vi "BuildCall.vi"(7 "PythonConverter_BD in":refnum<class "PyConvBD.lvclass">, 8 "error in":errorcluster, 11 "Constant in":refnum<class "Constant.lvclass">) -> (0 "error out":errorcluster, 3 "Constant out":refnum<class "Constant.lvclass">, 5 "PythonConverter_BD out":refnum<class "PyConvBD.lvclass">)   [LabVIEW 2014, in "Constant.lvclass"]
uses:
  Constant.lvclass
  Python/PythonConverter_BD/PyConvBD.lvclass
  Python/PythonConverter_BD/TypeDefs/NodeCall_TD.ctl
  Terminal/Terminal.lvclass
  Python/Parsing/Python Functions.lvlib
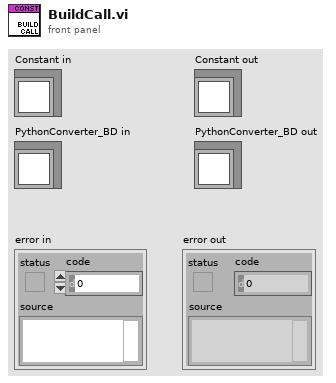
[diagram p1: front panel]
types:
  T1 = typedef "NodeCall_TD.ctl" = cluster{"call":string, "collect":string, "Threaded":bool, "branches":string[]}
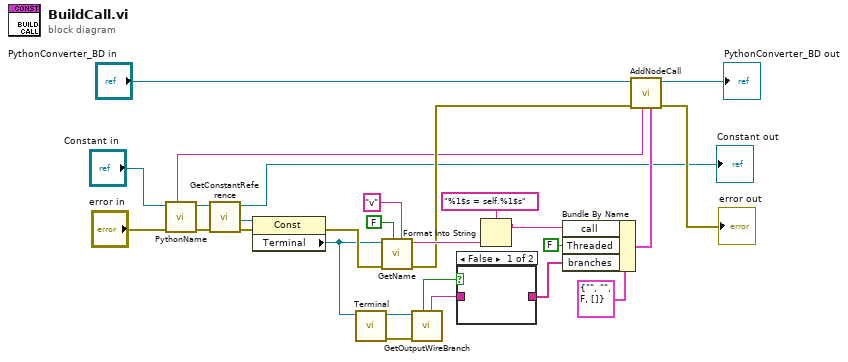
[diagram p0: block diagram]
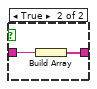
[diagram p2: hidden frame]
diagram:
  n1 = call-dynamic "PythonName.vi"("error in"="error in", "Constant in"="Constant in") -> ("error out"=w14:errorcluster, "Constant out"=w15:refnum<class "Constant.lvclass">, "UID"=w12:string)  [unwired: 6 in, 1 out]
  n2 = call "GetConstantReference.vi"("error in"=w14, "Constant in"=w15) -> ("error out"=w18:errorcluster, "reference out"=w17:refnum<vi>, "Constant out"=→"Constant out":refnum<class "Constant.lvclass">)  [unwired: 5 in]
  n3 = property class="Const"(reference=w17, error in=w18) -> (error out=w19:errorcluster, "Terminal"=w6:refnum<vi>)  [unwired: 1 out]
  n4 = call "Terminal.vi"("refnum"=w6) -> ("error out"=w4:errorcluster, "terminal"=w5:refnum<class "Terminal.lvclass">)  [unwired: 9 in]
  n5 = call "GetName.vi"("base name"="v", "add self"=FALSE, "error in"=w19, "GObj Refnum"=w6) -> ("error out"=w20:errorcluster, "name"=w23:string)  [unwired: 5 in, 1 out]
  n6 = call-dynamic "GetOutputWireBranch.vi"("error in"=w4, "Terminal in"=w5) -> ("branches"=w3:string, "branched"=w1:bool)  [unwired: 4 in, 2 out]
  n7 = case shown="False" w1 {
    tunnel: w3 -> [_ w29]
    tunnel: [_ w28] -> w2
    frame False {
    }
    frame True {
      n8 = Build Array(w29) -> (w28:string[])
    }
  }
  n9 = Format Into String(format string="%1$s = self.%1$s", w23) -> (resulting string=w9:string)  [unwired: 2 in, 1 out]
  n10 = Bundle By Name(cluster=T1 {"call"="", "collect"="", "Threaded"=FALSE, "branches"=[]} ("call"), "call"=w9, "Threaded"=FALSE, "branches"=w2) -> (w8:T1)
  n11 = call "AddNodeCall.vi"("call"=w8, "name"=w12, "error in"=w20, "PythonConverter_BD in"="PythonConverter_BD in") -> ("error out"=→"error out":errorcluster, "PythonConverter_BD out"=→"PythonConverter_BD out":refnum<class "PyConvBD.lvclass">)  [unwired: 4 in]
